vi "HoloPy_save_Features_csv.vi"(8 "error in (no error)":errorcluster, 9 "path csv file":path, 10 "Array":sgl[][](array[numeric]), 11 "Refnum in":refnum<k35>) -> (0 "error out":errorcluster, 3 "Refnum out":refnum<k35>)   [LabVIEW 2023, in "holoPyTracks.lvlib"]
uses:
  holoPyTracks.lvlib
panel:
  out "return value":string
  # "Python Node in holoPY.lvlib:HoloPy_Find_Features.vi->holoPY.lvlib:HoloPy_Example.vi<APPEND>\n\nPython returned the following error: Type mismatch while marshaling Python array. Expected type: float, received: void."
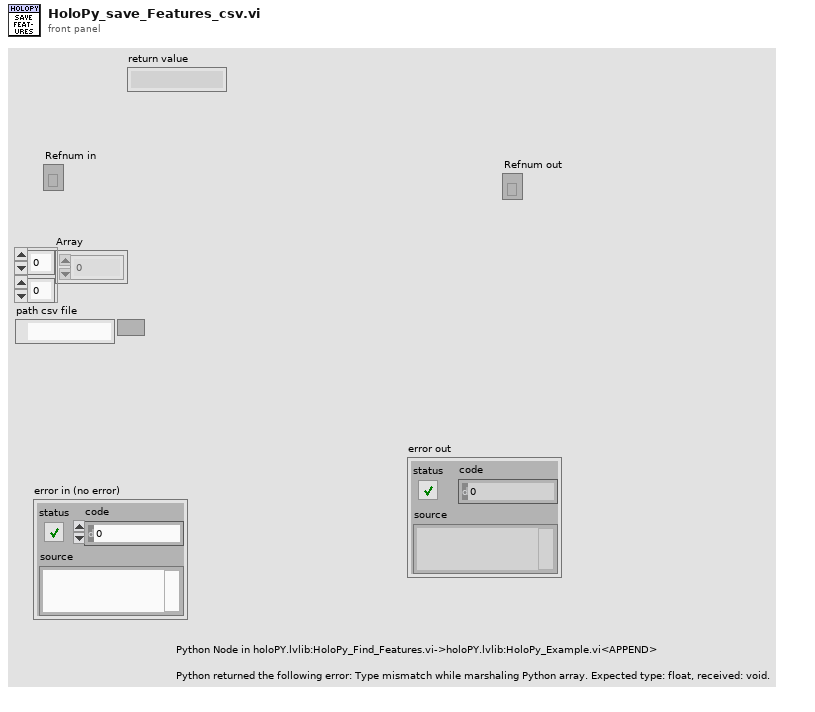
[diagram p1: front panel]
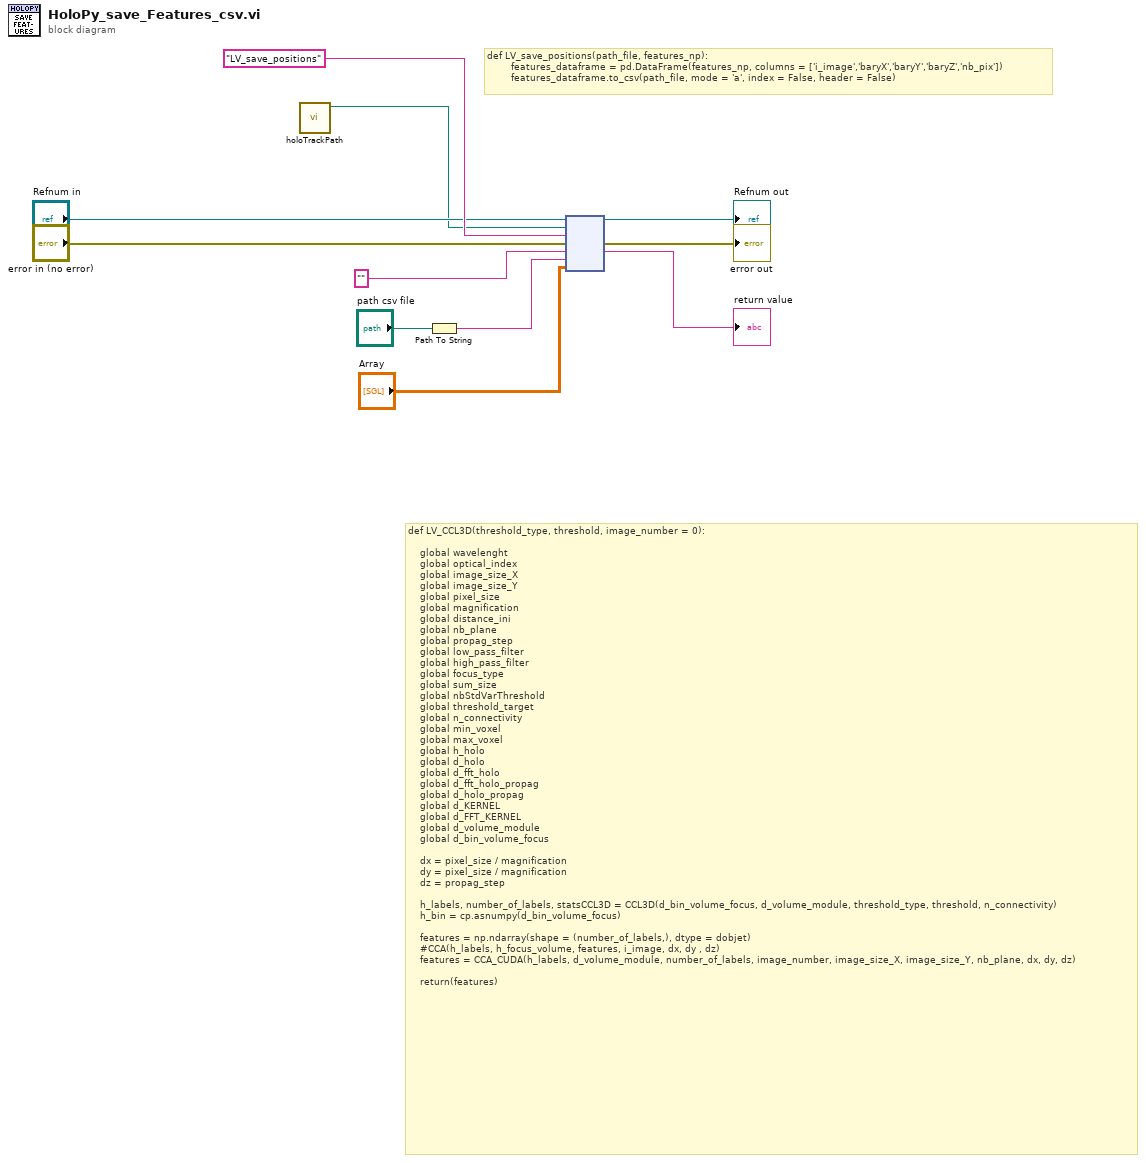
[diagram p0: block diagram]
diagram:
  # "def LV_save_positions(path_file, features_np):\n        features_dataframe = pd.DataFrame(features_np, columns = ['i_image','baryX','baryY','baryZ','nb_pix'])\n        features_dataframe.to_csv(path_file, mode = 'a', index = False, header = False)"
  # "def LV_CCL3D(threshold_type, threshold, image_number = 0):\n\n    global wavelenght \n    global optical_index \n    global image_size_X \n    global image_size_Y \n    global pixel_size \n    global magnification\n    global distance_ini\n    global nb_plane \n    global propag_step \n    global low_pass_filter\n    global high_pass_filter \n    global focus_type\n    global sum_size \n    global nbStdVarThreshold\n    global threshold_target\n    global n_connectivity\n    global min_voxel \n    global max_voxel\n    global h_holo\n    global d_holo\n    global d_fft_holo\n    global d_fft_holo_propag\n    global d_holo_propag\n    global d_KERNEL\n    global d_FFT_KERNEL\n    global d_volume_module\n    global d_bin_volume_focus\n\n    dx = pixel_size / magnification\n    dy = pixel_size / magnification\n    dz = propag_step\n\n    h_labels, number_of_labels, statsCCL3D = CCL3D(d_bin_volume_focus, d_volume_module, threshold_type, threshold, n_connectivity)\n    h_bin = cp.asnumpy(d_bin_volume_focus)\n\n    features = np.ndarray(shape = (number_of_labels,), dtype = dobjet)\n    #CCA(h_labels, h_focus_volume, features, i_image, dx, dy , dz)\n    features = CCA_CUDA(h_labels, d_volume_module, number_of_labels, image_number, image_size_X, image_size_Y, nb_plane, dx, dy, dz)\n\n    return(features)"
  n1 = call "holoTrackPath.vi"() -> ("appended path"=w6:path)  [unwired: 11 in]
  n2 = Path To String(path="path csv file") -> (string=w1:string)
  n3 = node("Refnum in", w6, "LV_save_positions" ("function name"), "error in (no error)", "", w1, "Array") -> (→"Refnum out":refnum<k35>, →"error out":errorcluster, →"return value":string)  [unwired: 2 in, 2 out]
